vi "Zaber A Series Commands and Responses.vi"() -> ()   [LabVIEW 2012]
doc: "This is a basic example demonstrating some of the basic read and write VIs, with some example commands and a variety of output formats displayed."
uses:
  <instrlib>/Zaber A Series/Zaber A Series.lvlib
panel:
  in  "Command":string
  out "Response Bundle Array":T1(array[cluster])
  out "First Response Data Value":string
  out "First Response Device Number":string
  out "Response String Array":string[](array[string])
  in  "VISA resource name":refnum<visa-resource-name>
  # "(c) 2014 Zaber Technologies.  ALL RIGHTS RESERVED."
  # "The purpose of this example is to show how you can enter commands and read back\nresponses. There are a number of ways to read responses, whether you just read one \nresponse, only want want part of the response, or prefer the complete string. Try writing\nsome of the example commands and see what response options are available. \n\nEnter the VISA resource your device is connected to and the Command string before running the VI."
  # "Example commands: \n'help' - view help info for device (view responses in String Array)\n'home' - device retracts to find the reference position\n'move rel 5000' - move the device by 5000 microsteps\n'01 get maxspeed' - returns the movement speed setting for device 1"
  # "If the command or data value you supply is not valid, you will get a warning message with a description of what the problem\nis in the error output."
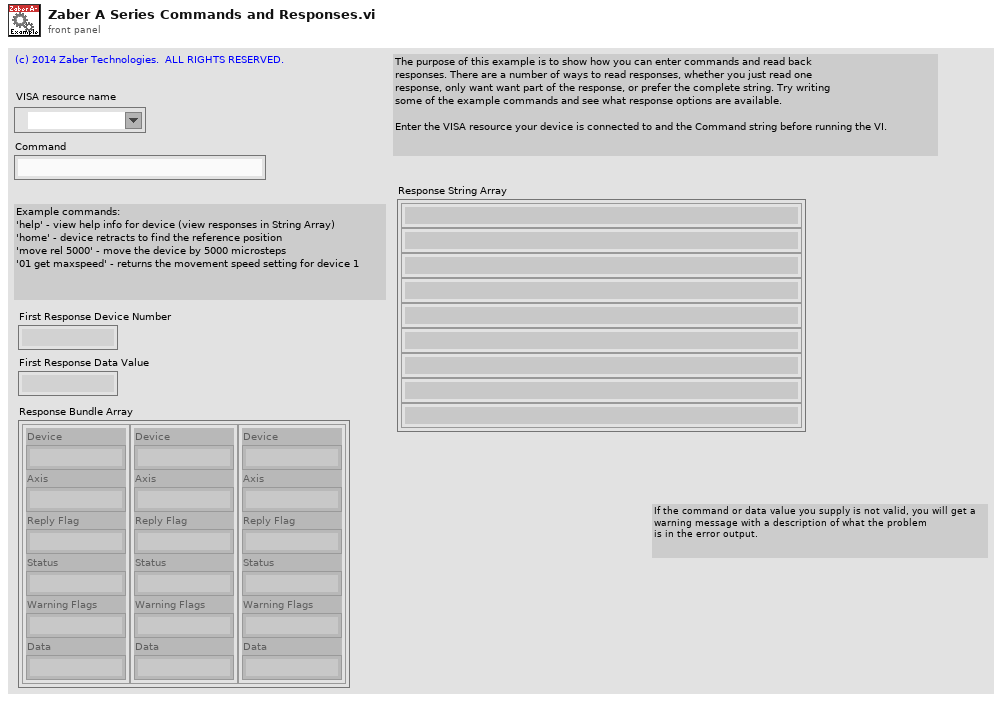
[diagram p1: front panel]
types:
  T1 = cluster{"Device":string, "Axis":string, "Reply Flag":string, "Status":string, "Warning Flags":string, "Data":string}[]
  T2 = cluster{"Device":string, "Axis":string, "Reply Flag":string, "Status":string, "Warning Flags":string, "Data":string}
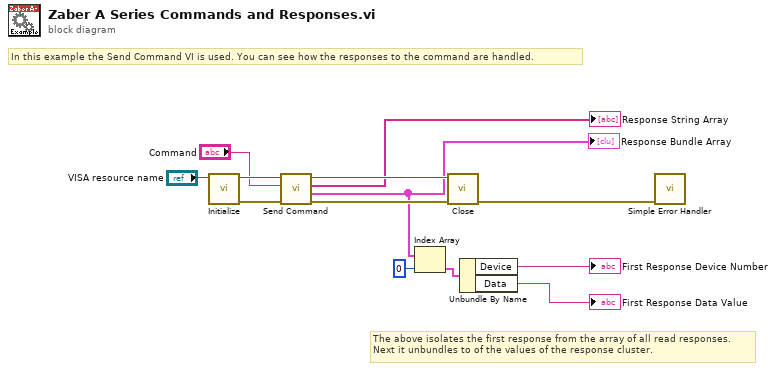
[diagram p0: block diagram]
diagram:
  # "In this example the Send Command VI is used. You can see how the responses to the command are handled."
  # "The above isolates the first response from the array of all read responses.\nNext it unbundles to of the values of the response cluster."
  n1 = call <instrlib>:"Initialize.vi"("VISA resource name"="VISA resource name") -> ("error out"=w6:errorcluster, "VISA resource name out"=w7:refnum<visa-resource-name>)  [unwired: 9 in]
  n2 = call <instrlib>:"Send Command.vi"("error in (no error)"=w6, "Command"="Command", "VISA resource name"=w7) -> ("error out"=w5:errorcluster, "Response Bundle Array"=w3:T1, "Response String Array"=→"Response String Array":string[], "VISA resource name out"=w4:refnum<visa-resource-name>)  [unwired: 4 in, 1 out]
  "Response Bundle Array" <- w3
  n3 = Index Array(array=w3, index=0) -> (element=w11:T2)
  n4 = call <instrlib>:"Close.vi"("error in (no error)"=w5, "VISA resource name"=w4) -> ("error out"=w8:errorcluster)  [unwired: 9 in]
  n5 = Unbundle By Name(w11) -> ("Device"=→"First Response Device Number":string, "Data"=→"First Response Data Value":string)
  n6 = call <vilib>:"Simple Error Handler.vi"("error in (no error)"=w8) -> ()  [unwired: 4 in, 5 out]
